vi "Get Page.vi"(8 "error in (no error)":errorcluster, 9 "Frame number":i32, 10 "Type of Image":T1(ring), 11 "TIFF File Ref":i32) -> (0 "error out":errorcluster, 1 "U16 Image out":u16[][](array[numeric]), 2 "I16 Image out":i16[][](array[numeric]), 3 "TIFF File Ref out":i32, 4 "Float32 Image out":sgl[][](array[numeric]), 5 "U8 Image out":u8[][](array[numeric]))   [LabVIEW 2012]
uses:
  VisualCPP/LabTIFF/Release/LabTIFF.dll
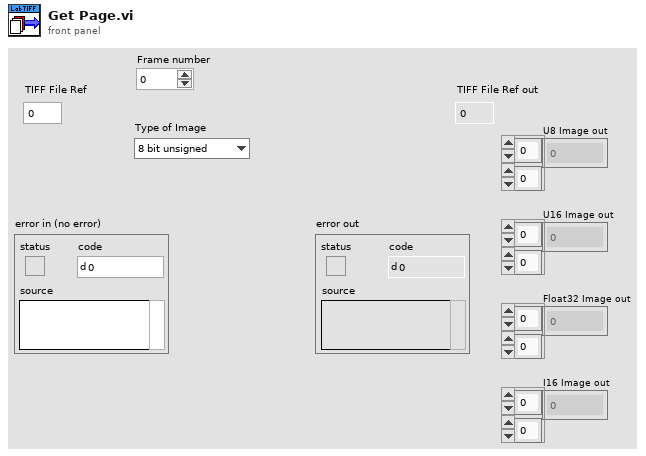
[diagram p1: front panel]
types:
  T1 = enum16{"8 bit unsigned", "16 bit unsigned", "16 bit signed", "32 bit float"}
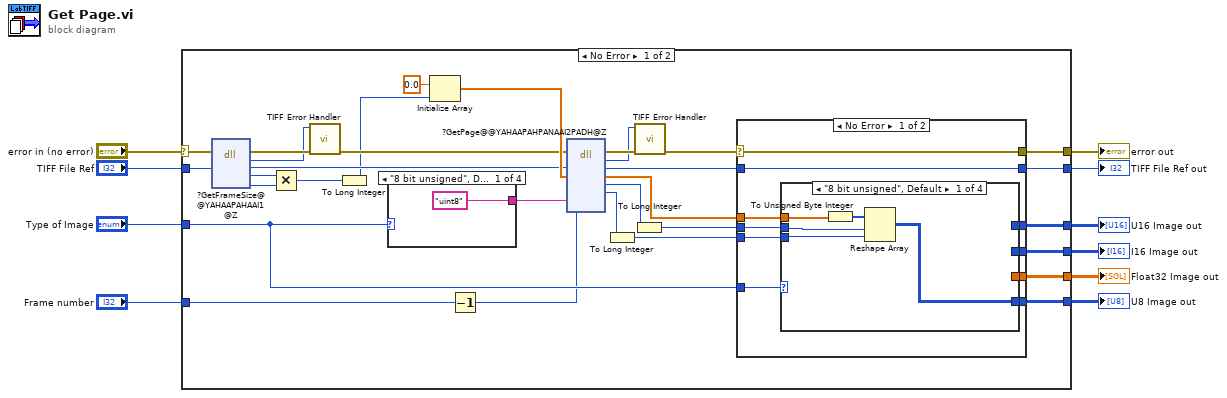
[diagram p0: block diagram]
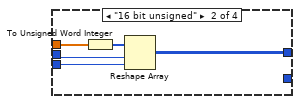
[diagram p2: hidden frame]
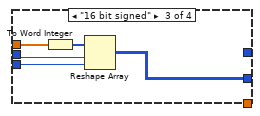
[diagram p3: hidden frame]
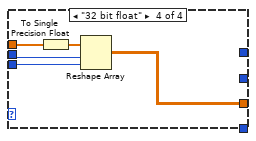
[diagram p4: hidden frame]
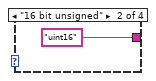
[diagram p6: hidden frame]
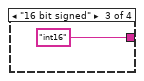
[diagram p7: hidden frame]
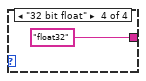
[diagram p8: hidden frame]
diagram:
  n1 = case shown="No Error" "error in (no error)" {
    selector: "error in (no error)" -> [w20 w79]
    tunnel: [w32 w79] -> w9
    tunnel: "TIFF File Ref" -> [w17 w78]
    tunnel: [w31 w78] -> w7
    tunnel: "Type of Image" -> [w37 _]
    tunnel: "Frame number" -> [w38 _]
    tunnel: [w27 _] -> w4
    tunnel: [w26 _] -> w3
    tunnel: [w25 _] -> w2
    tunnel: [w24 _] -> w1
    frame No Error {
      n2 = dll-call lib="C:/Users/Ludovico/Prog/moroder/dependencies/LabTIFF/VisualCPP/LabTIFF/Release/LabTIFF.dll" fn="?GetFrameSize@@YAHAAPAHAAI1@Z"(error in=w20, "FileRef"=w17) -> (error out=w19:errorcluster, "error"=w15:i32, "FileRef"=w16:i32, "ImageWidth"=w14:u32, "ImageHeight"=w13:u32)  [unwired: 4 in, 1 out]
      n3 = Multiply(x=w14, y=w13) -> (x*y=w12:u32)
      n4 = call "TIFF Error Handler.vi"("error in (no error)"=w19, "TIFF DLL error"=w15) -> ("error out"=w18:errorcluster)  [unwired: 9 in]
      n5 = To Long Integer(number=w12) -> (32bit integer=w11:i32)
      n6 = case shown="\"8 bit unsigned\", Default" w37 {
        tunnel: ["uint8" "uint16" "int16" "float32"] -> w39
        frame "8 bit unsigned", Default {
        }
        frame "16 bit unsigned" {
        }
        frame "16 bit signed" {
        }
        frame "32 bit float" {
        }
      }
      n7 = Initialize Array(0.0 ("element"), w11) -> (w21:dbl[])
      n8 = Decrement(x=w38) -> (x-1=w22:i32)
      n9 = dll-call lib="C:/Users/Ludovico/Prog/moroder/dependencies/LabTIFF/VisualCPP/LabTIFF/Release/LabTIFF.dll" fn="?GetPage@@YAHAAPAHPANAAI2PADH@Z"(error in=w18, "FileRef"=w16, "DataArray"=w21, "ImageType"=w39, "FrameIndex"=w22) -> (error out=w41:errorcluster, "return type"=w40:i32, "FileRef"=w30:i32, "DataArray"=w36:dbl[], "ImageHeight"=w35:u32, "ImageWidth"=w34:u32)  [unwired: 6 in, 1 out]
      n10 = To Long Integer(number=w34) -> (32bit integer=w28:i32)
      n11 = To Long Integer(number=w35) -> (32bit integer=w29:i32)
      n12 = call "TIFF Error Handler.vi"("error in (no error)"=w41, "TIFF DLL error"=w40) -> ("error out"=w33:errorcluster)  [unwired: 9 in]
      n13 = case shown="No Error" w33 {
        selector: w33 -> [w47 w73]
        tunnel: w37 -> [w51 _]
        tunnel: w36 -> [w50 _]
        tunnel: w29 -> [w49 _]
        tunnel: w28 -> [w48 _]
        tunnel: [w47 w73] -> w32
        tunnel: [w46 w72] -> w31
        tunnel: w30 -> [w46 w72]
        tunnel: [w45 _] -> w27
        tunnel: [w44 _] -> w26
        tunnel: [w43 _] -> w25
        tunnel: [w42 _] -> w24
        frame No Error {
          n14 = case shown="\"8 bit unsigned\", Default" w51 {
            tunnel: w50 -> [w54 w61 w66 w71]
            tunnel: w49 -> [w56 w59 w64 w69]
            tunnel: w48 -> [w55 w58 w63 w68]
            tunnel: [_ w57 _ _] -> w45
            tunnel: [_ _ w62 _] -> w44
            tunnel: [_ _ _ w67] -> w43
            tunnel: [w53 _ _ _] -> w42
            frame "8 bit unsigned", Default {
              n15 = To Unsigned Byte Integer(number=w54) -> (unsigned 8bit integer=w52:u8[])
              n16 = Reshape Array(w52, w56, w55) -> (w53:u8[][])
            }
            frame "16 bit unsigned" {
              n17 = To Unsigned Word Integer(number=w61) -> (unsigned 16bit integer=w60:u16[])
              n18 = Reshape Array(w60, w59, w58) -> (w57:u16[][])
            }
            frame "16 bit signed" {
              n19 = To Word Integer(number=w66) -> (16bit integer=w65:i16[])
              n20 = Reshape Array(w65, w64, w63) -> (w62:i16[][])
            }
            frame "32 bit float" {
              n21 = To Single Precision Float(number=w71) -> (single precision float=w70:sgl[])
              n22 = Reshape Array(w70, w69, w68) -> (w67:sgl[][])
            }
          }
        }
        frame Error {
        }
      }
    }
    frame Error {
    }
  }
  "error out" <- w9
  "TIFF File Ref out" <- w7
  "U16 Image out" <- w4
  "I16 Image out" <- w3
  "Float32 Image out" <- w2
  "U8 Image out" <- w1
